vi "mCodeGetPos.vi"() -> (1 "MCode get":string)   [LabVIEW 2014]
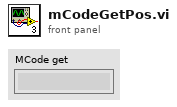
[diagram p1: front panel]
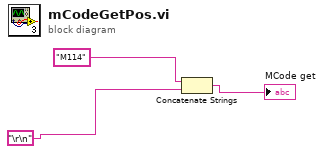
[diagram p0: block diagram]
diagram:
  n1 = Concatenate Strings("M114" ("String"), "\r\n") -> (→"MCode get":string)
